vi "MainBaxterDemo.vi"() -> ()   [LabVIEW 2012]
doc: "Demos several of Baxter's features: joint command, read joint states, open and close grippers, nod head, read IR data."
uses:
  <userlib>/ROSforLV/ROS/Code/JointPositions.ctl
  <userlib>/ROSforLV/ROS/Code/Slider.ctl
  <userlib>/ROSforLV/ROS/Code/SubVIs/BaxterSide.ctl
panel:
  in  "Mode":u8(ring)=1 items=["Position"=1, "Velocity"=2, "Effort"=3]
  out "Left Range Data":T1
  in  "Nod":bool
  in  "left gripper":u16(ring) items=["close"=0, "open"=100]
  in  "right gripper":u16(ring) items=["close"=0, "open"=100]
  in  "Parameters":T2 {"left_w2" scale=-180.0..180.0; "left_w1" scale=-180.0..180.0; "left_w0" scale=-180.0..180.0; "left_e1" scale=-180.0..180.0; "left_e0" scale=-180.0..180.0; "left_s1" scale=-180.0..180.0; "left_s0" scale=-180.0..180.0; "right_s1" scale=-180.0..180.0; "right_s0" scale=-180.0..180.0; "right_w2" scale=-180.0..180.0; "right_e1" scale=-180.0..180.0; "right_e0" scale=-180.0..180.0; "right_w0" scale=-180.0..180.0; "right_w1" scale=-180.0..180.0}
  out "Right Range Data":T1
  out "Joint States":T4(array[cluster])
  in  "disconnect head topic":bool
  in  "stop":bool
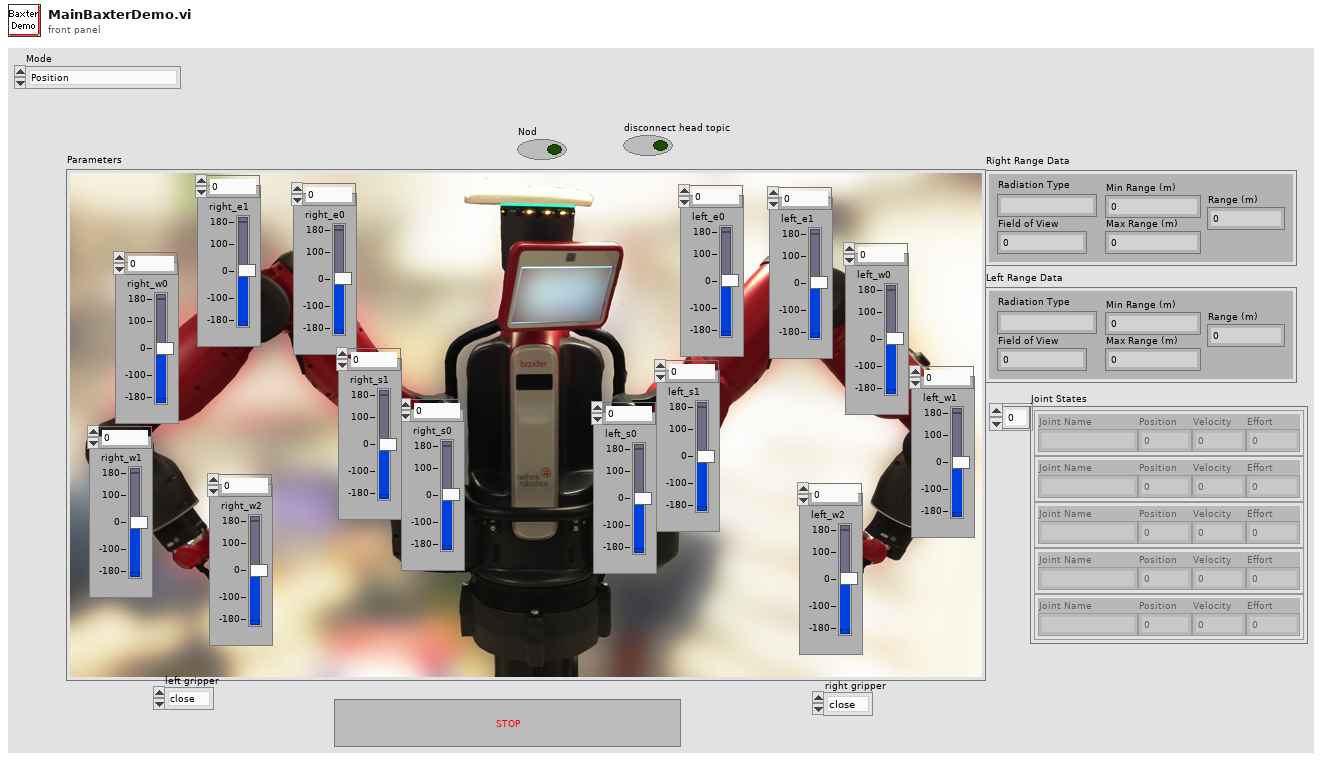
[diagram p1: front panel]
types:
  T1 = cluster{"Radiation Type":string, "Field of View":sgl, "Min Range (m)":sgl, "Max Range (m)":sgl, "Range (m)":sgl}
  T2 = typedef "JointPositions.ctl" = cluster{"left_e0":T3, "left_e1":T3, "left_s0":T3, "left_s1":T3, "left_w0":T3, "left_w1":T3, "left_w2":T3, "right_e0":T3, "right_e1":T3, "right_s0":T3, "right_s1":T3, "right_w0":T3, "right_w1":T3, "right_w2":T3}
  T3 = typedef "Slider.ctl" = dbl
  T4 = cluster{"Joint Name":string, "Position":dbl, "Velocity":dbl, "Effort":dbl}[]
  T5 = typedef "BaxterSide.ctl" = enum16{"left", "right"}
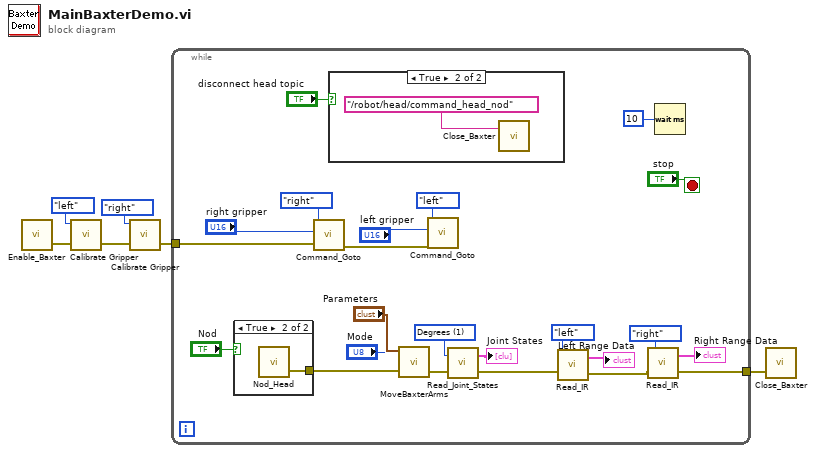
[diagram p0: block diagram]
diagram:
  n1 = call <userlib>:"Enable_Baxter.vi"() -> ("error out"=w5:errorcluster)  [unwired: 4 in]
  n2 = call <userlib>:"Calibrate Gripper.vi"("Side"=BaxterSide."left", "error in"=w5) -> ("error out"=w6:errorcluster)  [unwired: 4 in]
  n3 = call <userlib>:"Calibrate Gripper.vi"("Side"=BaxterSide."right", "error in"=w6) -> ("error out"=w4:errorcluster)  [unwired: 4 in]
  n4 = while {
    tunnel: [w26] -> w1
    tunnel: w4 -> [w21]
    stop <- "stop" stop-if-true
    w22 = u16 1 items=["Radians", "Degrees"] ("Units (Rad)")
    n5 = case shown="True" "Nod" {
      tunnel: [_ w31] -> w23
      frame False {
      }
      frame True {
        n6 = call <userlib>:"Nod_Head.vi"() -> ("error out"=w31:errorcluster)  [unwired: 4 in]
      }
    }
    n7 = call <userlib>:"Command_Goto.vi"("Side"=BaxterSide."right", "Desired Position"="right gripper", "error in"=w21) -> ("error out"=w19:errorcluster)  [unwired: 3 in]
    n8 = case shown="True" "disconnect head topic" {
      frame False {
      }
      frame True {
        n9 = call <userlib>:"Close_Baxter.vi"("topic"="/robot/head/command_head_nod") -> ()  [unwired: 3 in, 1 out]
      }
    }
    n10 = call <userlib>:"MoveBaxterArms.vi"("Parameters"="Parameters", "Mode"="Mode", "error in"=w23) -> ("error out"=w18:errorcluster)  [unwired: 3 in]
    n11 = call <userlib>:"Command_Goto.vi"("Side"=BaxterSide."left", "Desired Position"="left gripper", "error in"=w19) -> ()  [unwired: 3 in, 1 out]
    n12 = call <userlib>:"Read_Joint_States.vi"("error in"=w18, "Units (deg)"=w22) -> ("error out"=w11:errorcluster, "Joint States"=→"Joint States":T4)  [unwired: 1 in]
    n13 = call <userlib>:"Read_IR.vi"("error in"=w11, "Side"=BaxterSide."left") -> ("error out"=w10:errorcluster, "Range Data"=→"Left Range Data":T1)  [unwired: 1 in]
    n14 = call <userlib>:"Read_IR.vi"("error in"=w10, "Side"=BaxterSide."right") -> ("error out"=w26:errorcluster, "Range Data"=→"Right Range Data":T1)  [unwired: 1 in]
    n15 = Wait (ms)(milliseconds to wait=u32 10) -> ()  [unwired: 1 out]
  }
  n16 = call <userlib>:"Close_Baxter.vi"("error in"=w1) -> ()  [unwired: 3 in, 1 out]
